vi "error graph.vi"() -> (3 "Yerror":dbl[](array[numeric]), 5 "Y error bars":T3(graph))   [LabVIEW 2016]
doc: "This VI allows for the addition of error bars to a XY scatter plot in X, Y or both directions.\n\nThe mandatory XY plot input should contain the plot to which error bars are to be added; the Xerror and Yerror inputs contain the point by point error in these scatter plot points.\n\nThe outputs are in the XY scatter plot data type, which can readily be appended to an existing plot.\n\n\n© 2007, VU University Amsterdam\nJoost van Mameren, jmameren@gmail.com"
uses:
  controls/data control cluster.ctl
panel:
  in  "error in":errorcluster
  out "error out":errorcluster
  in  "DATA CLUSTER out":T1
  out "Numeric":i32
  out "Cycle data by seq":dbl[][][](array[numeric])
  out "Yerror 2":dbl[](array[numeric])
  out "output cluster":T2
  out "Cluster":cluster{dbl[], dbl[]}
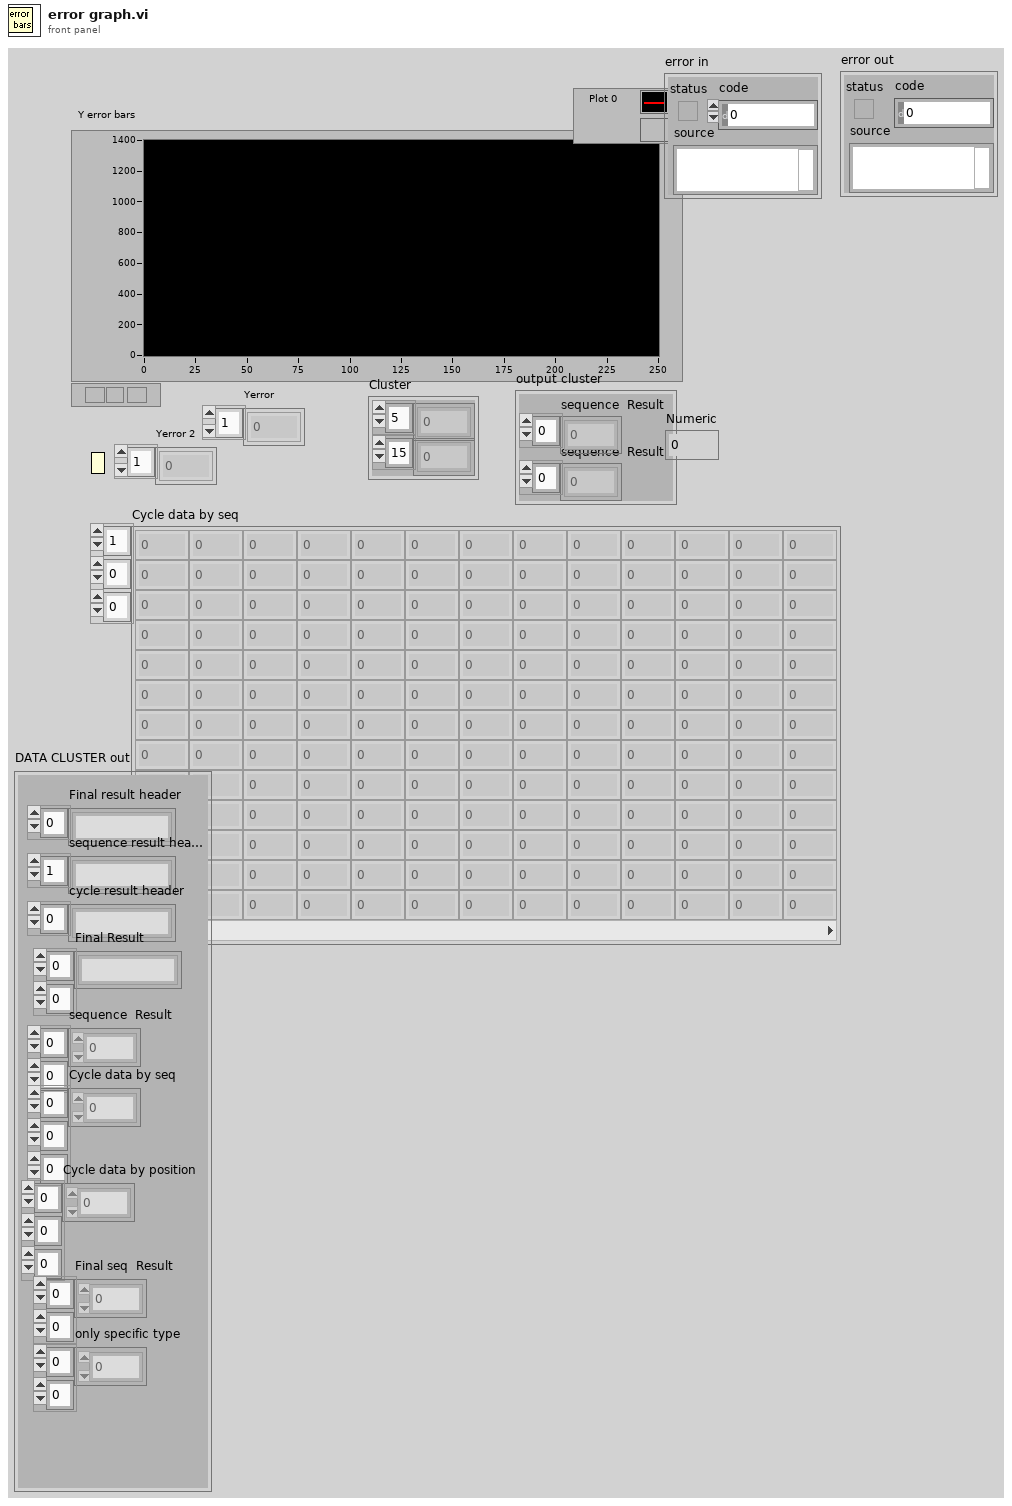
[diagram p1: front panel]
types:
  T1 = typedef "data control cluster.ctl" = cluster{"Final result header":string[], "sequence result header":string[], "cycle result header ":string[], "Final Result":string[][], "sequence  Result":dbl[][], "Cycle data by seq":dbl[][][], "Cycle data by position":dbl[][][], "Final seq  Result":dbl[][], "only specific type":dbl[][]}
  T2 = cluster{"sequence  Result":dbl[], "sequence  Result":dbl[]}
  T3 = cluster{"sequence  Result":dbl[], "sequence  Result":dbl[]}[]
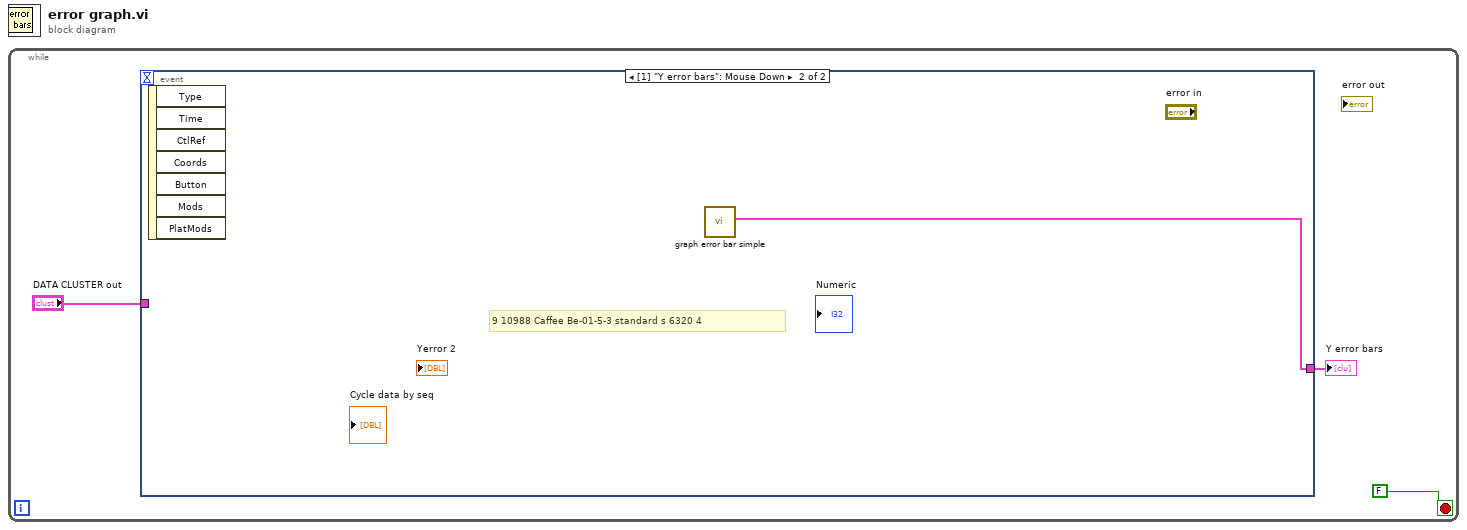
[diagram p0: block diagram]
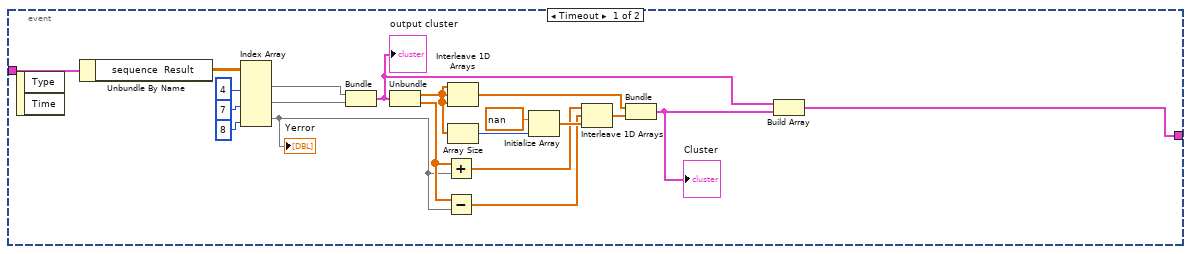
[diagram p2: hidden frame]
diagram:
  # "9\t10988\tCaffee\tBe-01-5-3 standard\ts\t6320\t4"
  n1 = while {
    stop <- FALSE ("stop") stop-if-true
    n2 = event shown="[1] \"Y error bars\": Mouse Down" {
      selector: _ -> [_ _]
      dyn-events: _ -> [_ _]
      timeout: _ -> [_ _]
      tunnel: "DATA CLUSTER out" -> [w21 _]
      tunnel: [w4 w24] -> w2
      event Timeout {
        n3 = event-data() -> ()  [unwired: 1 in, 2 out]
        n4 = Unbundle By Name(w21) -> ("sequence  Result"=w20:dbl[][])
        n5 = Index Array(array=w20, index (col) #1=4 ("disabled index (col)"), index (col) #2=7 ("index (col)"), index (col) #3=8 ("index (col)")) -> (element #1=w15:dbl[], element #2=w14:dbl[], element #3=w16:dbl[])  [unwired: 3 in]
        "Yerror" <- w16
        n6 = Bundle("sequence  Result"=w15, "sequence  Result"=w14) -> (w13:T2)  [unwired: 1 in]
        "output cluster" <- w13
        n7 = Unbundle(w13) -> ("sequence  Result"=w23:dbl[], "sequence  Result"=w22:dbl[])
        n8 = Add(x=w22, y=w16) -> (x+y=w7:dbl[])
        n9 = Subtract(x=w22, y=w16) -> (x-y=w8:dbl[])
        n10 = Interleave 1D Arrays(w23, w23, w23) -> (w6:dbl[])
        n11 = Array Size(array=w23) -> (size(s)=w9:i32)
        n12 = Initialize Array(nan ("element"), w9) -> (w10:dbl[])
        n13 = Interleave 1D Arrays(w7, w8, w10) -> (w5:dbl[])
        n14 = Bundle(w6, w5) -> (w12:cluster{dbl[], dbl[]})  [unwired: 1 in]
        "Cluster" <- w12
        n15 = Build Array(w13, w12) -> (w4:T3)
      }
      event "Y error bars": Mouse Down {
        n16 = event-data() -> ()  [unwired: 1 in, 7 out]
        n17 = call "graph error bar simple.vi"() -> ("graph out"=w24:T3)  [unwired: 10 in, 1 out]
      }
    }
    "Y error bars" <- w2
  }
